vi "simulation of servo has integrator.vi"() -> ()   [LabVIEW 2021]
uses:
  <vilib>/addons/Control Design/_Model Construction/Model Typedefs.llb/CD State Space Model (MIMO).ctl
  <vilib>/addons/Control Design/_Model Construction/Model Typedefs.llb/CD General Elements.ctl
  <vilib>/Analysis/Matrix/Datatypes/RealMatrix.ctl
  <vilib>/Simulation/Scripting/Companion Diagram/SimConfigNode/SimParams.ctl
  <vilib>/Simulation/Scripting/Companion Diagram/SimConfigNode/_simSolvers.ctl
  <vilib>/Simulation/Implementation/Shared/SIMSCR Execution Mode.ctl
  <vilib>/Simulation/Param Hierarchy/Typedefs/SIMPH Param Control Actions.ctl
  <vilib>/Simulation/Implementation/Shared/NILVSim_ParamChanged.vi
  <vilib>/Simulation/Implementation/Shared/NILVSIM_BeginStep.vi
  <vilib>/Simulation/DataSources/Implementation/NILVSim Step.llb/SIM Step (scalar).vi
  <vilib>/Simulation/ContinuousLinear/Implementation/NILVSim State Space.llb/SIM State Space Distributor (CD).vi
  <vilib>/Simulation/SignalArithmetic/Implementation/NILVSim Gain.llb/SIM Gain (vector,MatrixGain).vi
  <vilib>/Simulation/SignalDisplay/Implementation/NILVSim Time Waveform.llb/SIM Time Waveform (vector).vi
  <vilib>/Simulation/SignalArithmetic/Implementation/NILVSim Gain.llb/SIM Gain (vector,ScalarGain).vi
  <vilib>/Simulation/ContinuousLinear/Implementation/NILVSim State Space.llb/SIM State Space Collector (CD).vi
  <vilib>/Simulation/Implementation/Shared/NILVSim_Manager.vi
  <vilib>/Utility/error.llb/Clear Errors.vi
  <vilib>/Simulation/Implementation/Shared/NILVSim_FinalizeModel.vi
  <vilib>/addons/Control Design/_Model Construction/Model Creation.llb/Model Creation SubVI/cd_Create State Space Model.vi
  <vilib>/addons/Control Design/_Time Response Analysis/Time Response.llb/Time Response subVI/cd_Step Response (State-Space).vi
  <vilib>/addons/Control Design/_Dynamic Analysis/Dynamic Analysis.llb/Dynamic Analysis subVI/cd_Poles (State-Space).vi
  <vilib>/addons/Control Design/_Dynamic Analysis/Dynamic Analysis.llb/Dynamic Analysis subVI/cd_Pole-Zero Map (State-Space).vi
  <vilib>/addons/Control Design/_Utility/Model Viewer.llb/Model Viewer SubVI/cd_Draw State-Space Equation (SS).vi
  <vilib>/Analysis/baseanly.llb/Real Inverse Matrix.vi
  <vilib>/Simulation/Implementation/Shared/SIM Unbundle Sim Info.vi
  <vilib>/Simulation/Implementation/Shared/NILVSim_Initialize.vi
  <vilib>/Simulation/Utility/Implementation/NILVSim Get Time and IsAcceptedStep.vi
  <vilib>/Simulation/Implementation/Shared/SIMSH Read Queue.vi
  <vilib>/Simulation/Implementation/Shared/NILVSim_GetModelError.vi
  <vilib>/Simulation/Implementation/Shared/SIM Bundle Sim Info.vi
  <vilib>/Simulation/Scripting/Companion Diagram/SimConfigNode/SimDog.xnode
  <vilib>/Simulation/Implementation/XNodeFramework/SimXNode/SimX.xnode
  <vilib>/addons/Control Design/_Model Construction/NI_LinSys_Model Creation.lvlib
  <vilib>/addons/Control Design/_State-Space Analysis/NI_CD_State-Space Analysis.lvlib
  <vilib>/addons/Control Design/_Utility/NI_CD_Model Viewer.lvlib
  <vilib>/Analysis/NI_AALBase.lvlib
  <vilib>/addons/Control Design/_State Feedback Control/NI_CD_State Feedback Control.lvlib
  <vilib>/addons/Control Design/_Dynamic Analysis/NI_CD_Dynamic Analysis.lvlib
  <vilib>/addons/Control Design/_Model Construction/NI_LinSys_Model Typedefs.lvlib
  <vilib>/Simulation/ContinuousLinear/Implementation/NILVSim State Space.llb/SIM State Space (CD).vi
  <vilib>/addons/Control Design/_Time Response Analysis/NI_CD_Time Response.lvlib
  <vilib>/Simulation/Implementation/Shared/NI_SIM_Implementation.lvlib
  <vilib>/Analysis/Matrix/NI_Matrix.lvlib
panel:
  out "control Action u":waveform(dbl)[](graph)=[{"t0"=timestamp(10 s since 1904-01-01), "dt"=1.0, "Y"=[-6.137394897556069e-07]}]
  out "Step Response uncompansated":cluster{"time":dbl[], dbl[]}[](graph)=[{"time"=[0.0, 0.006272421747822789, 0.012544843495645578, 0.018817265243468367, 0.025089686991291157, 0.03136210873911394, 0.03763453048693673, 0.04390695223475952, 0.05017937398258231, 0.056451795730405104, 0.06272421747822789, 0.06899663922605068, 0.07526906097387347, 0.08154148272169626, 0.08781390446951905, 0.09408632621734184, 0.10035874796516463, 0.10663116971298742, 0.11290359146081021, 0.119176013208633, 0.12544843495645577, 0.13172085670427858, 0.13799327845210135, 0.14426570019992416, 0.15053812194774693, 0.15681054369556974, 0.1630829654433925, 0.16935538719121532, 0.1756278089390381, 0.1819002306868609, 0.18817265243468367, 0.19444507418250648, 0.20071749593032925, 0.20698991767815203, 0.21326233942597483, 0.2195347611737976, 0.22580718292162041, 0.2320796046694432, 0.238352026417266, 0.24462444816508877, 0.25089686991291155, 0.2571692916607344, 0.26344171340855715, 0.26971413515637993, 0.2759865569042027, 0.28225897865202554, 0.2885314003998483, 0.2948038221476711, 0.30107624389549387, 0.30734866564331664, 0.3136210873911395, 0.31989350913896225, 0.326165930886785, 0.3324383526346078, 0.33871077438243063, 0.3449831961302534, 0.3512556178780762, 0.35752803962589896, 0.3638004613737218, 0.37007288312154457, 0.37634530486936735, 0.3826177266171901, 0.38889014836501296, 0.39516257011283573, 0.4014349918606585, 0.4077074136084813, 0.41397983535630406, 0.4202522571041269, 0.42652467885194967, 0.43279710059977244, 0.4390695223475952, 0.44534194409541805, 0.45161436584324083, 0.4578867875910636, 0.4641592093388864, 0.4704316310867092, 0.476704052834532, 0.48297647458235476, 0.48924889633017754, 0.4955213180780004, 0.5017937398258231, 0.5080661615736459, 0.5143385833214688, 0.5206110050692915, 0.5268834268171143, 0.533155848564937, 0.5394282703127599, 0.5457006920605827, 0.5519731138084054, 0.5582455355562282, 0.5645179573040511, 0.5707903790518738, 0.5770628007996966, 0.5833352225475193, 0.5896076442953422, 0.595880066043165, 0.6021524877909877, 0.6084249095388106, 0.6146973312866333, 0.6209697530344561, 0.627242174782279], [0.0, 9.835858149863949e-06, 3.9343906683652405e-05, 8.852556810530234e-05, 0.00015738321409266572, 0.0002459201667549117, 0.00035414070039382233, 0.000482050043769917, 0.0006296543828746048, 0.0007969608642098375, 0.0009839775985769988, 0.0011907136653770407, 0.0014171791174241468, 0.0016633849862754725, 0.0019293432880797916, 0.0022150670299481458, 0.0025205702168498772, 0.0028458678590376997, 0.0031909759800057454, 0.003555911624984806, 0.003940692869979272, 0.004345338831350558, 0.004769869675952105, 0.005214306631821324, 0.005678671999434143, 0.006162989163528149, 0.006667282605500566, 0.007191577916387654, 0.0077359018104324155, 0.00830028213924779, 0.008884747906582861, 0.009489329283699891, 0.010114057625370338, 0.01075896548649834, 0.011424086639380488, 0.012109456091611013, 0.012815110104641913, 0.013541086213007824, 0.01428742324422586, 0.015054161339380957, 0.015841341974407633, 0.016649007982079446, 0.01747720357471784, 0.018325974367632336, 0.01919536740330462, 0.020085431176329223, 0.020996215659124105, 0.02192777232842473, 0.022880154192575705, 0.023853415819634412, 0.024847613366301594, 0.02586280460769417, 0.026899048967976097, 0.027956407551863537, 0.02903494317702098, 0.030134720407365527, 0.031255805587297035, 0.032398266876872174, 0.033562174287941116, 0.034747599721266016, 0.03595461700464092, 0.03718330193203335, 0.03843373230376829, 0.03970598796777591, 0.04100015086192489, 0.042316305057463685, 0.043654536803592964, 0.04501493457319271, 0.04639758910972821, 0.047802593475359915, 0.049230043100282554, 0.05068003583331977, 0.052152671993801025, 0.053648054424748286, 0.05516628854740075, 0.05670748241710643, 0.05827174678061029, 0.05985919513476934, 0.06146994378672566, 0.06310411191556951, 0.06476182163552488, 0.06644319806069138, 0.06814836937137643, 0.0698774668820532, 0.07163062511098003, 0.07340798185151863, 0.07520967824518845, 0.07703585885649633, 0.07888667174958079, 0.08076226856671186, 0.08266280460868777, 0.08458843891717152, 0.08653933435901057, 0.08851565771258461, 0.0905175797562272, 0.09254527535876794, 0.0945989235722434, 0.09667870772682588, 0.09878481552802028, 0.10091743915618073, 0.10307677536839963]}]
  out "[0 K2 K3 K4 ....]":dbl[][](array[numeric])=[[0.0, -1394.064816326529, -282.64489795918354, -280.51591836734667]]
  out "K1":dbl=-1013.5510204081628
  in  "r(t)":dbl=0.1
  out "Waveform Chart":waveform(dbl)[](graph)=[{"t0"=timestamp(10 s since 1904-01-01), "dt"=1.0, "Y"=[0.09999999898834172]}, {"t0"=timestamp(10 s since 1904-01-01), "dt"=1.0, "Y"=[0.1]}]
  out "Open Loop Poles":cdb[](array[numeric])=[3.6708309685955305+0.0i, -3.67083096859553+0.0i, 0.0+0.0i, 0.0+0.0i] format="%.3f"
  out "Pole-Zero Map":cluster{dbl[], dbl[]}[](graph)=[{[3.6708309685955305, -3.67083096859553, 0.0, 0.0], [0.0, 0.0, 0.0, 0.0]}, {[-3.5, 3.500000000000001], [0.0, 0.0]}]
  out "K (Gain)":dbl[][](array[numeric])=[[-1013.5510204081628, -1394.064816326529, -282.64489795918354, -280.51591836734667]] format="%.2f"
  in  "Gain Type":u16(ring) items=["Controller Gain", "Observer Gain (Predictive)", "Observer Gain (Current)"]
  in  "Desired Poles":cdb[](array[numeric])=[-2.0+5.2i, -2.0-5.2i, -10.0+0.0i, -20.0+0.0i] format="%.2f"
  out "Transformation Matrix(T)":T1=[[-6.125000000000001, -2.220446049250313e-16, 0.5, 1.7765721119653683e-33], [1.3288986138578397e-47, 2.7755575615628914e-16, -0.625, -2.2207151399567104e-33], [-2.7200464103316367e-16, -6.125000000000001, -2.2204460492503128e-16, 0.5], [3.740063814205997e-15, 0.0, 2.7755575615628914e-16, -0.625]]
  out "Equation":picture
  in  "Form Type":u16(ring)=1 items=["Modal"=0, "Companion"=5, "Controllability"=1, "Controller Companion"=2, "Observability"=3, "Observer Companion"=4]
  out "Transformation Matrix inverse (T')":dbl[][](array[numeric])=[[-0.16326530612244897, -0.13061224489795917, 0.0, 0.0], [-7.250436079184695e-17, -5.800348863347757e-17, -0.16326530612244897, -0.13061224489795917], [-3.2198404294735173e-32, -1.6, -7.250436079184695e-17, -5.800348863347756e-17], [-9.769962616701378e-16, -1.4921397450962105e-15, -3.2198404294735173e-32, -1.6]] format="%.2f"
  out "new Transformed Model":T2={"properties"={"Model name"="System Model", "Input names"=["u0"], "Output names"=["y0"], "Input Delays"=[0.0], "Output Delays"=[0.0], "Sampling Time"=0.0, "Notes"=""}, "A"=[[-4.4408920985006257e-16, 0.9999999999999999, 1.5407439555097887e-33, -3.469446951953614e-18], [-1.9721522630525295e-31, 5.7777898331617076e-34, 0.9999999999999999, 6.162975822039155e-33], [-5.984102102729594e-15, 2.565854121688508e-49, -9.918539213594265e-32, 1.0], [-5.3149503489265676e-30, 2.98904327368899e-31, 13.475000000000001, 4.440892098500626e-16]], "B"=[[0.0], [-3.469446951953614e-18], [-1.5407439555097887e-33], [1.0]], "C"=[[-6.125, -2.220446049250313e-16, 0.5, 0.0]], "D"=[[0.0]], "StateNames"=["x0", "x1", "x2", "x3"], "Transport Delay"=[[0.0]]} {"Transport Delay" format="%.2f"; "D" format="%#.2g"; "C" format="%#.2g"; "B" format="%#.2g"; "A" format="%#.2g"; "properties"."Sampling Time" format="%#.6p"; "properties"."Output Delays" format="%.4f"; "properties"."Input Delays" format="%.4f"}
  out "Is Controllable?":bool=TRUE
  out "Controllability Matrix (M)":dbl[][](array[numeric])=[[0.0, 0.5, 0.0, 0.6125], [0.0, -0.625, 0.0, -8.421875], [0.5, 0.0, 0.6125, 0.0], [-0.625, 0.0, -8.421875, 0.0]] format="%.2f"
  in  "D":dbl[][](array[numeric])=[[0.0]] format="%#.5g"
  in  "C":dbl[][](array[numeric])=[[1.0, 0.0, 0.0, 0.0]] format="%#.5g"
  in  "B":dbl[][](array[numeric])=[[0.0], [0.0], [0.5], [-0.625]] format="%#.5g"
  in  "A":dbl[][](array[numeric])=[[0.0, 0.0, 1.0, 0.0], [0.0, 0.0, 0.0, 1.0], [0.0, -0.98, 0.0, 0.0], [0.0, 13.475, 0.0, 0.0]] format="%#.5g"
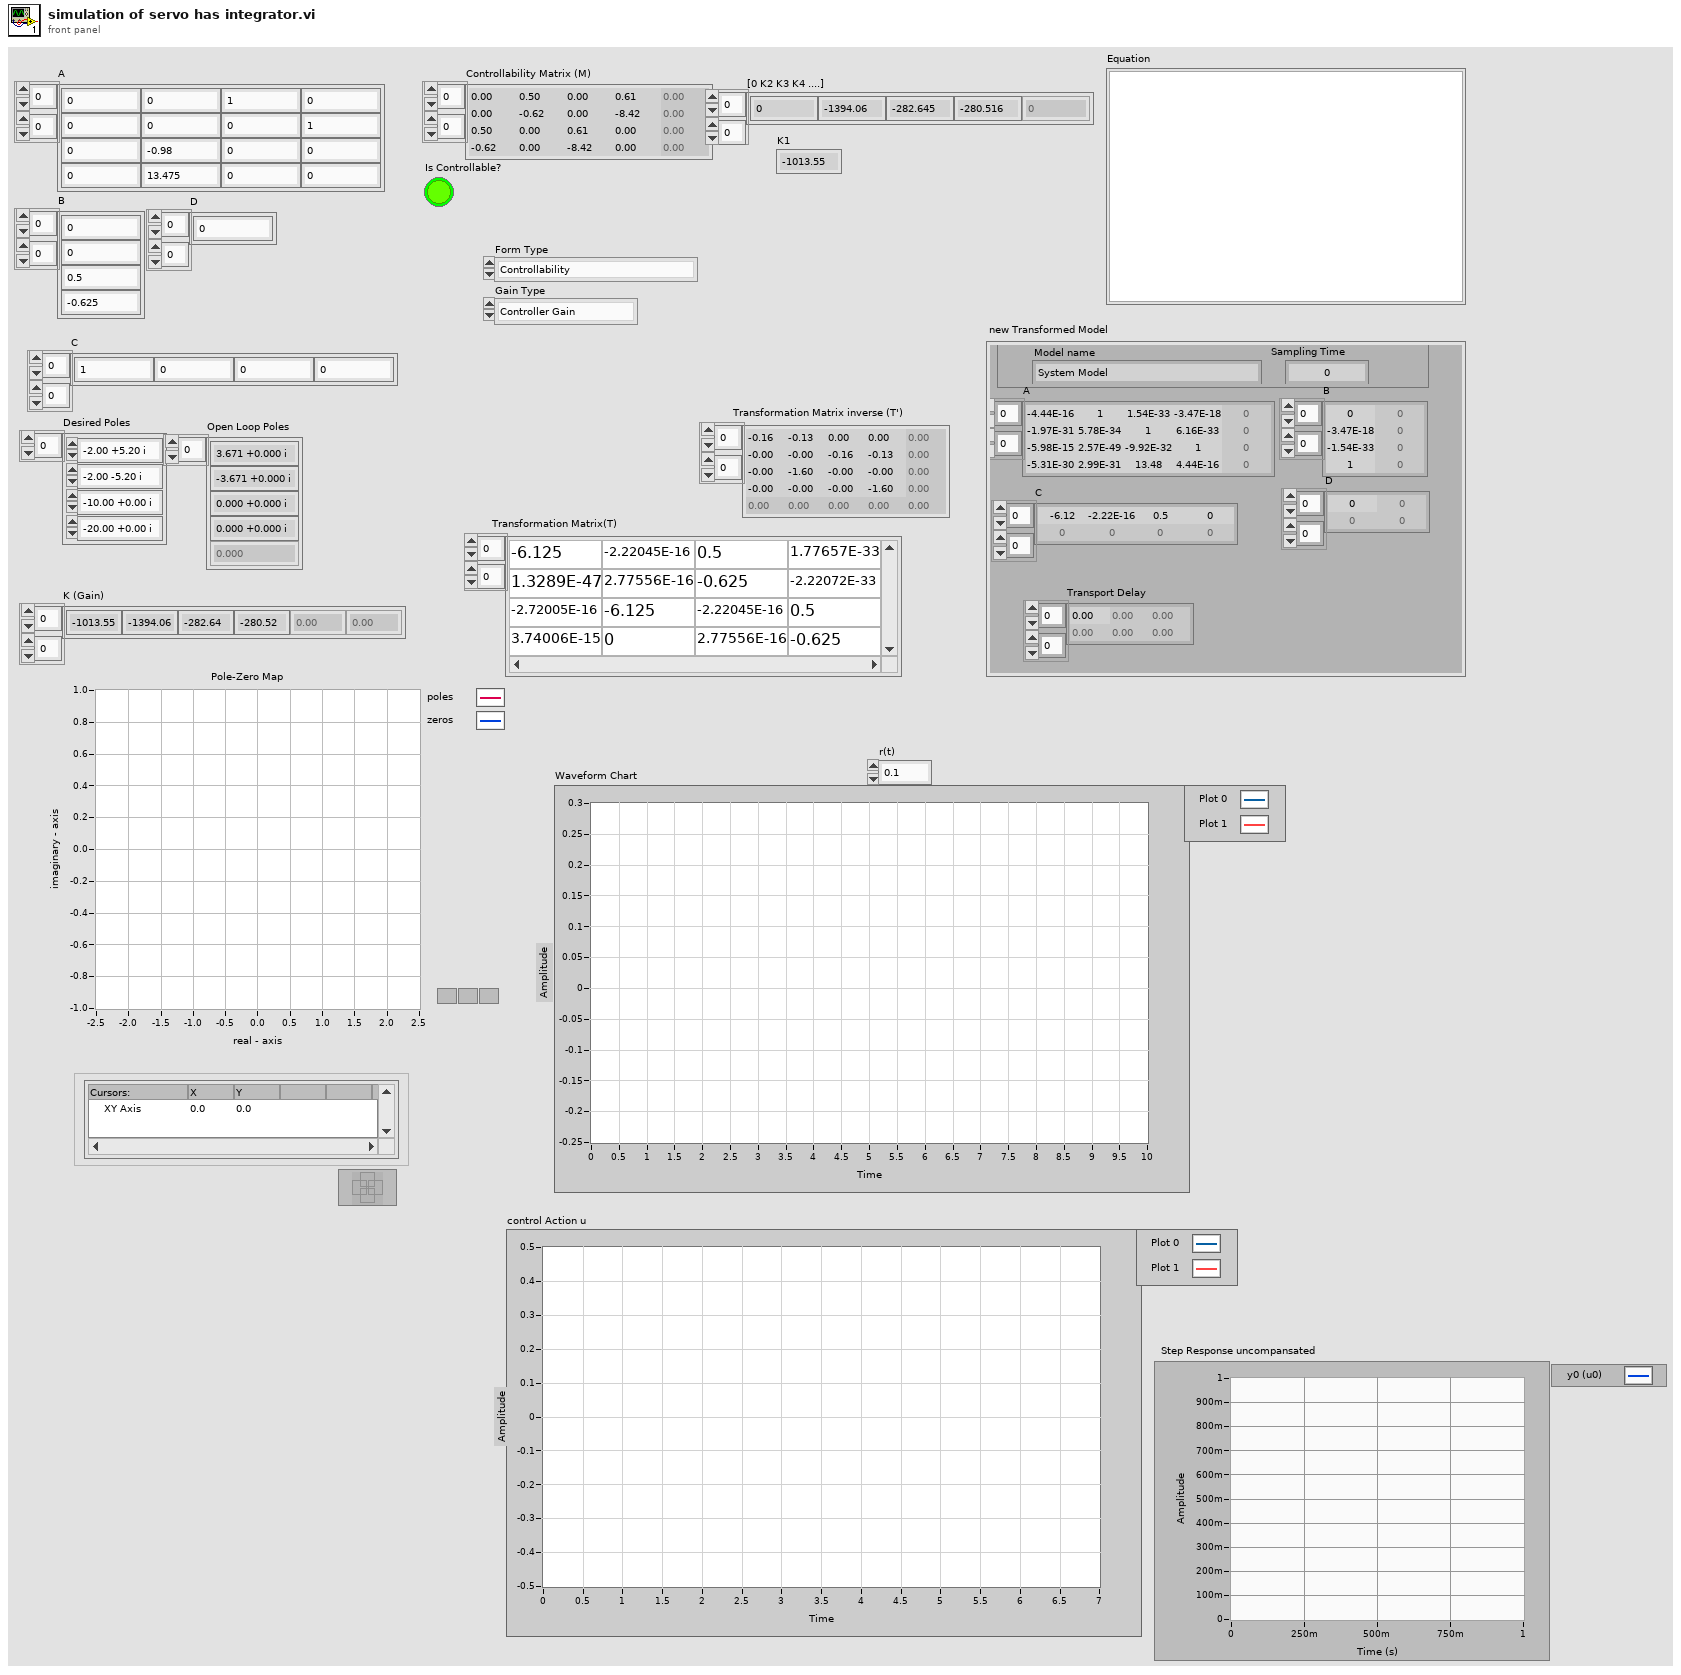
[diagram p1: front panel]
types:
  T1 = typedef "NI_Matrix.lvlib/RealMatrix.ctl" = dbl[][]
  T2 = typedef "NI_LinSys_Model Typedefs.lvlib/CD State Space Model (MIMO).ctl" = cluster{"properties":T3, "A":dbl[][], "B":dbl[][], "C":dbl[][], "D":dbl[][], "StateNames":string[], "Transport Delay":dbl[][]}
  T3 = typedef "NI_LinSys_Model Typedefs.lvlib/CD General Elements.ctl" = cluster{"Model name":string, "Input names":string[], "Output names":string[], "Input Delays":dbl[], "Output Delays":dbl[], "Sampling Time":dbl, "Notes":string}
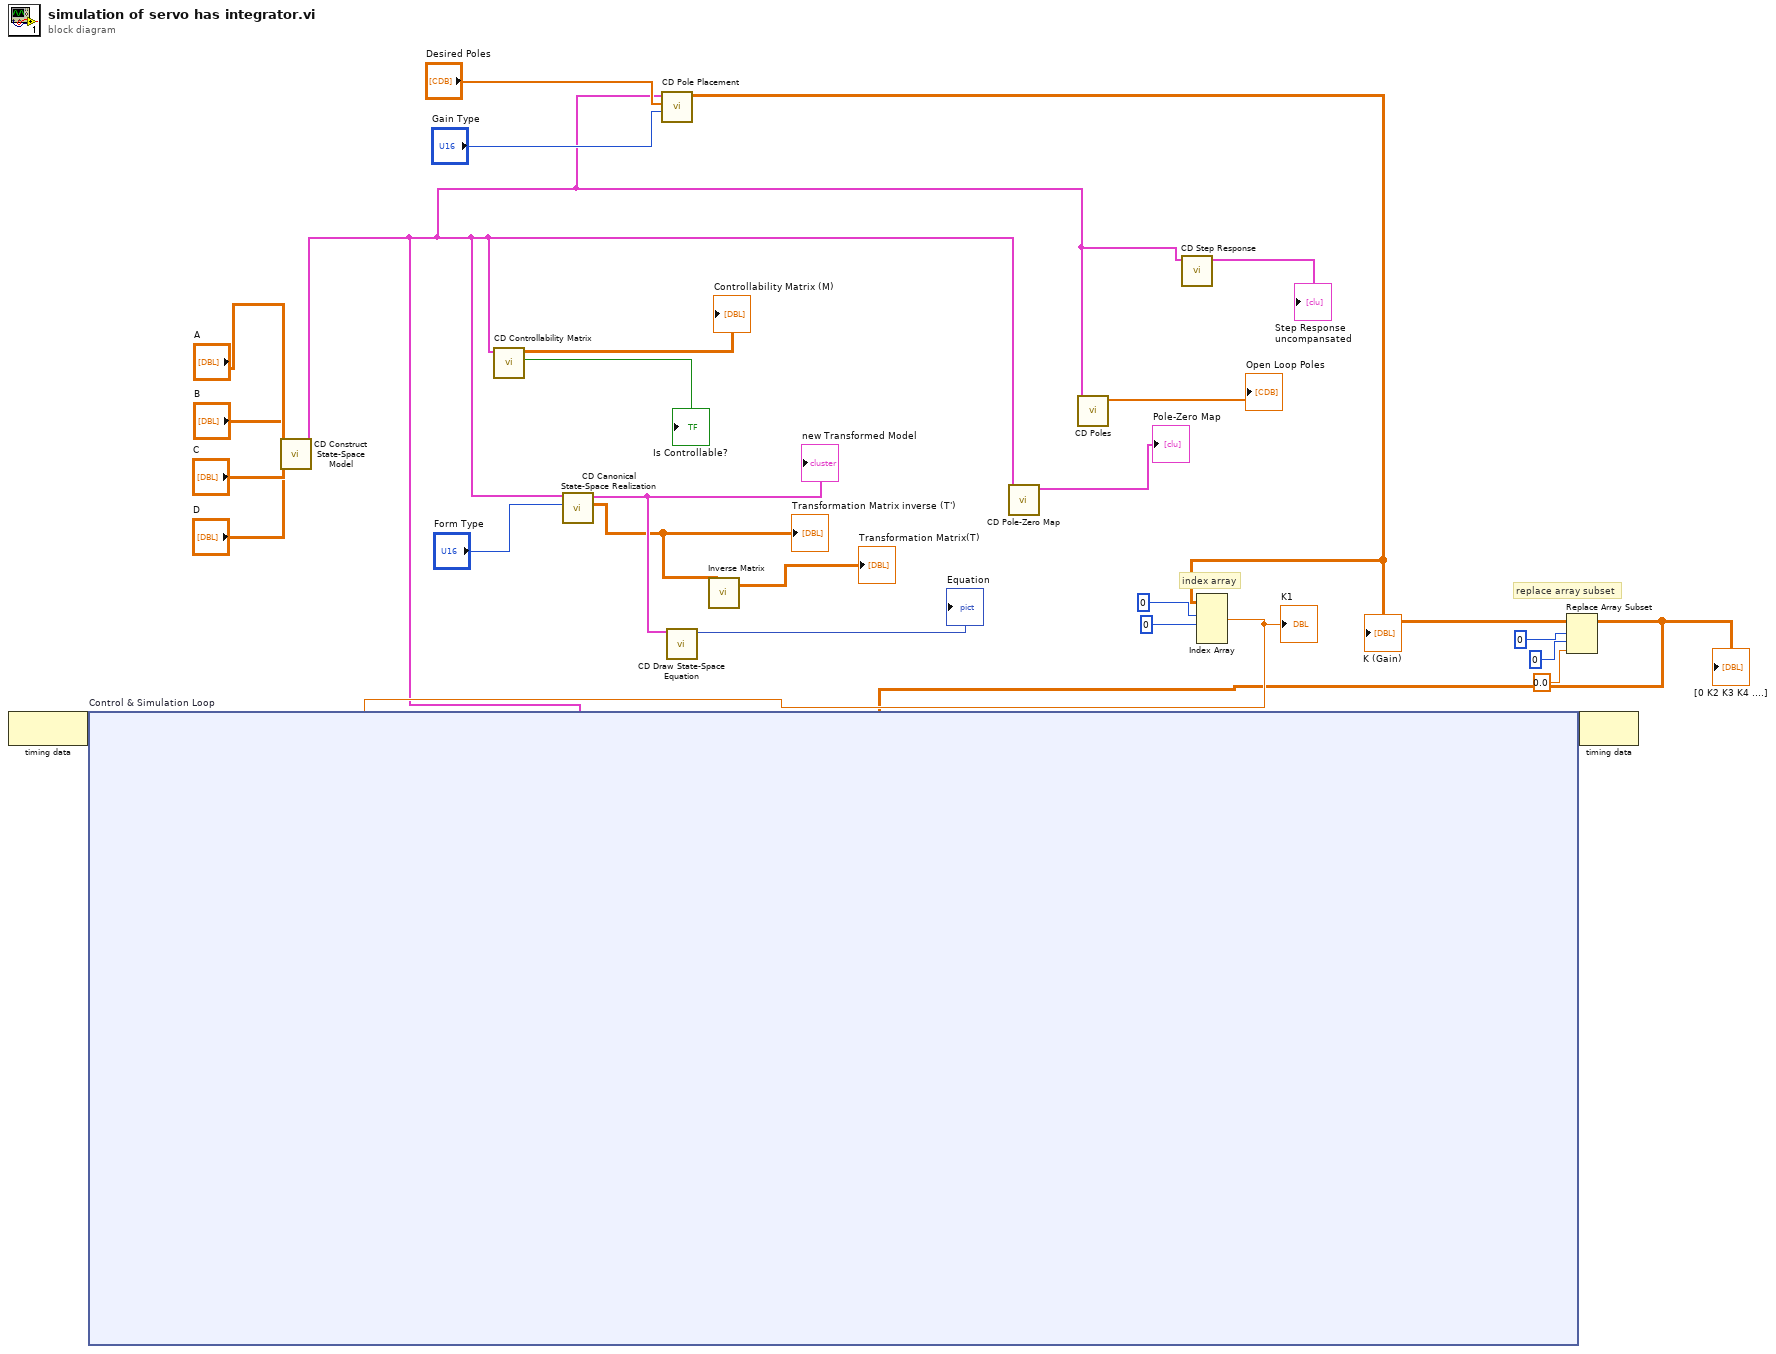
[diagram p0: block diagram]
diagram:
  # "index array"
  # "replace array subset"
  n1 = node-c288() -> (w12:variant)  [unwired: 1 in]
  n2 = call-poly <vilib>:"CD Construct State-Space Model.vi"("A"="A", "B"="B", "C"="C", "D"="D") -> ("State-Space Model"=w2:T2)  [unwired: 10 in, 1 out]
  n3 = call <vilib>:"CD Controllability Matrix.vi"("State-Space Model"=w2) -> ("Is Controllable?"=→"Is Controllable?":bool, "Controllability Matrix"=→"Controllability Matrix (M)":dbl[][])  [unwired: 7 in, 2 out]
  n4 = call <vilib>:"CD Canonical State-Space Realization.vi"("Form Type"="Form Type", "State-Space Model"=w2) -> ("Transformation Matrix (T)"=w22:dbl[][], "Transformed Model"=w24:T2)  [unwired: 7 in, 1 out]
  "new Transformed Model" <- w24
  "Transformation Matrix inverse (T')" <- w22
  n5 = call <vilib>:"CD Pole Placement.vi"("Gain Type"="Gain Type", "Poles"="Desired Poles", "State-Space Model"=w2) -> ("Gain"=w7:dbl[][])  [unwired: 6 in, 2 out]
  "K (Gain)" <- w7
  n6 = call-poly <vilib>:"CD Draw State-Space Equation.vi"("State-Space Model"=w24) -> ("Equation"=→"Equation":picture)  [unwired: 8 in, 2 out]
  n7 = call-poly <vilib>:"Inverse Matrix.vi"("Input Matrix"=w22) -> ("Inverse Matrix"=→"Transformation Matrix(T)":T1)  [unwired: 1 in, 1 out]
  n8 = call-poly <vilib>:"CD Pole-Zero Map.vi"("State-Space Model"=w2) -> ("Pole-Zero Map"=→"Pole-Zero Map":cluster{dbl[], dbl[]}[])  [unwired: 7 in, 3 out]
  n9 = call-poly <vilib>:"CD Poles.vi"("State-Space Model"=w2) -> ("Poles"=→"Open Loop Poles":cdb[])  [unwired: 9 in, 1 out]
  n10 = call-poly <vilib>:"CD Step Response.vi"("State-Space Model"=w2) -> ("Step Response Graph"=→"Step Response uncompansated":cluster{"time":dbl[], dbl[]}[])  [unwired: 7 in, 3 out]
  n11 = Index Array(array=w7, index (row) #1=0 ("index (row)"), index (col) #1=0 ("disabled index (col)")) -> (element #1=w9:dbl)  [unwired: 2 in, 1 out]
  "K1" <- w9
  n12 = Replace Array Subset(array=w7, new element=0.0 ("new element/subarray"), index (row)=0, index (col)=0 ("disabled index (col)")) -> (w3:dbl[][])
  "[0 K2 K3 K4 ....]" <- w3
  n13 = node-c254 "Control & Simulation Loop"(w12, w2, w9, w3) -> (w11:variant)
  n14 = node-c288(w11) -> ()  [unwired: 1 out]
